vi "Step_Dir_to_CW_CCW.vi"(7 "invert":bool, 10 "step":bool, 11 "direction":bool) -> (2 "CCW":bool, 3 "CW":bool)   [LabVIEW 2014]
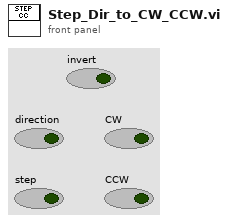
[diagram p1: front panel]
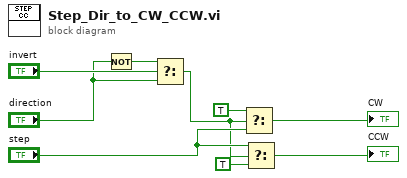
[diagram p0: block diagram]
diagram:
  n1 = Not(x="direction") -> (.not. x?=w5:bool)
  n2 = Select(t=w5, s="invert", f="direction") -> (s? t:f=w3:bool)
  n3 = Select(t=TRUE, s=w3, f="step") -> (s? t:f=→"CW":bool)
  n4 = Select(t="step", s=w3, f=TRUE) -> (s? t:f=→"CCW":bool)
